vi "34970 Initialize +++.vi"(0 "VISA resource name":refnum<visa-resource-name>, 5 "ID Query (T: Check)":bool=TRUE, 7 "Instr Config":enum16{"no change", "Reset", "Preset"}(ring), 9 "Serial Port Configuration":T1={"Timeout Value (10000)"=10000, "Baud Rate (57600)"=enum."57600", "Flow Control (1:XON / XOFF)"=enum."XON / XOFF"}, 11 "error in (no error)":errorcluster) -> (4 "VISA session":refnum<visa-resource-name>, 15 "error out":errorcluster)   [LabVIEW 2020]
doc: "This VI passes the addressing information for GPIB, or the serial port configuration to the VISA Open VI. You must run this VI before using any of the instrument driver VIs for this instrument.\n\nIt can optionally check the the instrument ID, but error reporting for this still flawed. Modified to allow instrument configuration Reset, Preset(see pp 160, 161 user manual), or No Change.\nW. Gilbert, University of Minnesota Physics, 8/6/2004\nwgilbert@physics.umn.edu"
panel:
  # "See 34970 manual\npp 160,161"
  # "Check\nDon't Check"
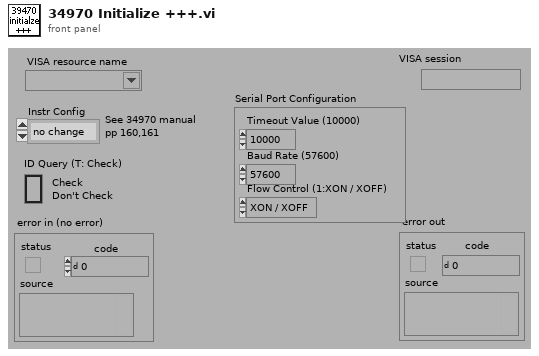
[diagram p1: front panel]
types:
  T1 = cluster{"Timeout Value (10000)":u32, "Baud Rate (57600)":enum16{"1200", "2400", "4800", "9600", "19200", "38400", "57600", "115200"}, "Flow Control (1:XON / XOFF)":enum16{"None", "XON / XOFF", "RTS / CTS", "DTR / DSR"}}
  T2 = enum16{"1200", "2400", "4800", "9600", "19200", "38400", "57600", "115200"}
  T3 = enum16{"None", "XON / XOFF", "RTS / CTS", "DTR / DSR"}
  T4 = cluster{"status":bool, "code":i32, "VI Name":string}
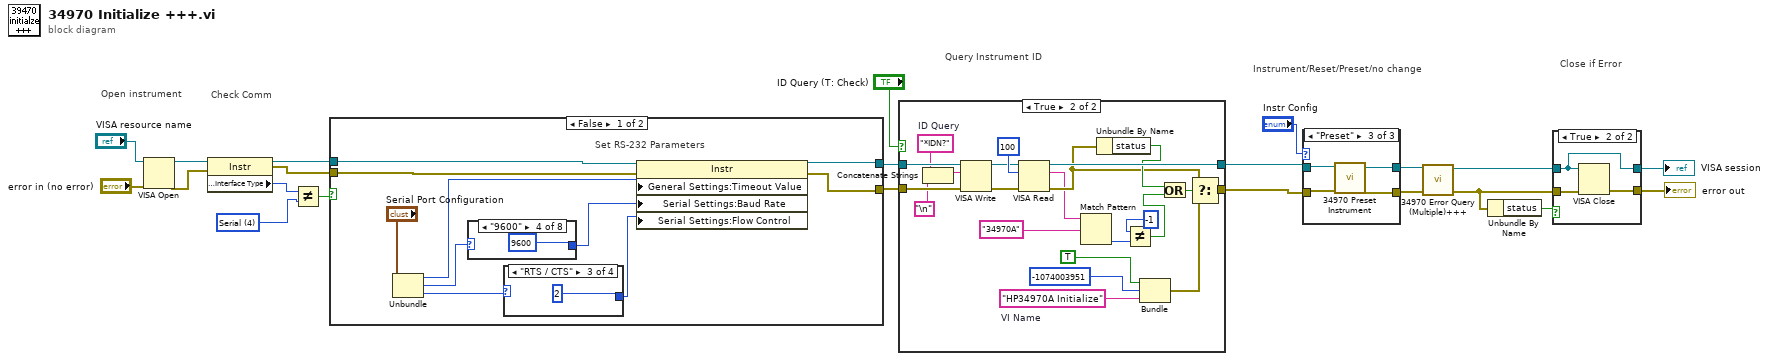
[diagram p0: block diagram]
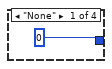
[diagram p2: hidden frame]
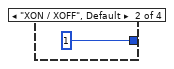
[diagram p3: hidden frame]
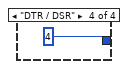
[diagram p4: hidden frame]
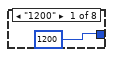
[diagram p5: hidden frame]
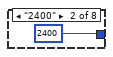
[diagram p6: hidden frame]
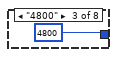
[diagram p7: hidden frame]
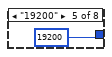
[diagram p8: hidden frame]
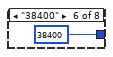
[diagram p9: hidden frame]
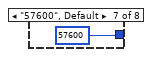
[diagram p10: hidden frame]
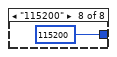
[diagram p11: hidden frame]
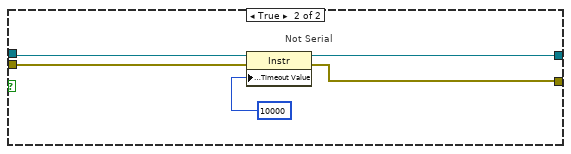
[diagram p12: hidden frame]
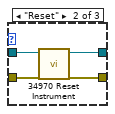
[diagram p15: hidden frame]
diagram:
  w13 = u16 4 items=["GPIB"=1, "VXI"=2, "GPIB-VXI"=3, "Serial"=4, "PXI"=5] ("Interface Information:Interface Type")
  # "Check Comm"
  # "Close if Error"
  # "Query Instrument ID"
  # "Instrument/Reset/Preset/no change"
  # "Open instrument"
  n1 = VISA Open(error in (no error)="error in (no error)", VISA resource name="VISA resource name") -> (VISA resource name=w17:refnum<visa-resource-name>, error out=w14:errorcluster)  [unwired: 1 in, 2 out]
  n2 = property class="Instr"(reference=w17, error in=w14) -> (reference out=w16:refnum<visa-resource-name>, error out=w15:errorcluster, "Interface Information:Interface Type"=w10:u16)
  n3 = Not Equal?(x=w10, y=w13) -> (x != y?=w12:bool)
  n4 = case shown="False" w12 {
    tunnel: [w24 w47] -> w9
    tunnel: w16 -> [w32 w49]
    tunnel: [w23 w45] -> w8
    tunnel: w15 -> [w31 w48]
    frame False {
      # "Set RS-232 Parameters"
      n5 = Unbundle("Serial Port Configuration") -> ("Timeout Value (10000)"=w27:u32, "Baud Rate (57600)"=w29:T2, "Flow Control (1:XON / XOFF)"=w26:T3)
      n6 = case shown="\"9600\"" w29 {
        tunnel: [u32 1200 u32 2400 u32 4800 u32 9600 u32 19200 u32 38400 u32 57600 u32 115200] -> w28
        frame "1200" {
        }
        frame "2400" {
        }
        frame "4800" {
        }
        frame "9600" {
        }
        frame "19200" {
        }
        frame "38400" {
        }
        frame "57600", Default {
        }
        frame "115200" {
        }
      }
      n7 = case shown="\"RTS / CTS\"" w26 {
        tunnel: [0 1 2 4] -> w25
        frame "None" {
        }
        frame "XON / XOFF", Default {
        }
        frame "RTS / CTS" {
        }
        frame "DTR / DSR" {
        }
      }
      n8 = property class="Instr"(reference=w32, error in=w31, "General Settings:Timeout Value"=w27, "Serial Settings:Baud Rate"=w28, "Serial Settings:Flow Control"=w25) -> (reference out=w24:refnum<visa-resource-name>, error out=w23:errorcluster)
    }
    frame True {
      # "Not Serial"
      n9 = property class="Instr"(reference=w49, error in=w48, "General Settings:Timeout Value"=u32 10000 ("Tmo Value")) -> (reference out=w47:refnum<visa-resource-name>, error out=w45:errorcluster)
    }
  }
  n10 = case shown="True" "ID Query (T: Check)" {
    tunnel: [w50 w73] -> w5
    tunnel: [w51 w70] -> w6
    tunnel: w9 -> [w51 w71]
    tunnel: w8 -> [w50 w72]
    frame False {
    }
    frame True {
      w52 = "*IDN?"  # ID Query
      w55 = "HP34970A Initialize"  # VI Name
      n11 = Concatenate Strings(w52, "\n") -> (w53:string)
      n12 = VISA Write(VISA resource name=w71, write buffer=w53, error in (no error)=w72) -> (VISA resource name out=w58:refnum<visa-resource-name>, error out=w60:errorcluster)  [unwired: 1 out]
      n13 = VISA Read(VISA resource name=w58, byte count=u32 100, error in (no error)=w60) -> (VISA resource name out=w70:refnum<visa-resource-name>, read buffer=w57:string, error out=w59:errorcluster)  [unwired: 1 out]
      n14 = Match Pattern(string=w57, regular expression="34970A") -> (offset past match=w65:i32)  [unwired: 4 out]
      n15 = Unbundle By Name(w59) -> ("status"=w62:bool)
      n16 = Not Equal?(x=-1, y=w65) -> (x != y?=w56:bool)
      n17 = Bundle(TRUE, -1074003951, "VI Name"=w55) -> (w67:cluster{bool, i32, "VI Name":string})  [unwired: 1 out]
      n18 = Or(x=w62, y=w56) -> (x .or. y?=w61:bool)
      n19 = Select(t=w59, s=w61, f=w67) -> (s? t:f=w73:T4)
    }
  }
  n20 = case shown="\"Preset\"" "Instr Config" {
    tunnel: w5 -> [w74 w76 w82]
    tunnel: [w74 w79 w80] -> w3
    tunnel: w6 -> [w75 w77 w83]
    tunnel: [w75 w78 w81] -> w4
    frame "no change", Default {
    }
    frame "Reset" {
      n21 = call "34970 Reset Instrument.vi"("VISA resource name"=w77, "error in (no error)"=w76) -> ("VISA resource name out"=w78:refnum<visa-resource-name>, "error out"=w79:errorcluster)  [unwired: 12 in]
    }
    frame "Preset" {
      n22 = call "34970 Preset Instrument.vi"("error in (no error)"=w82, "VISA session"=w83) -> ("error out"=w80:errorcluster, "dup VISA session"=w81:refnum<visa-resource-name>)  [unwired: 8 in]
    }
  }
  n23 = call "34970 Error Query (Multiple)+++.vi"("VISA resource name"=w4, "error in (no error)"=w3) -> ("VISA resource name out"=w2:refnum<visa-resource-name>, "error out"=w1:errorcluster)  [unwired: 10 in, 2 out]
  n24 = Unbundle By Name(w1) -> ("status"=w19:bool)
  n25 = case shown="True" w19 {
    tunnel: w2 -> [w85 w86]
    tunnel: w1 -> [w84 w88]
    tunnel: [w85 w86] -> w18
    tunnel: [w84 w87] -> w11
    frame False {
    }
    frame True {
      n26 = VISA Close(VISA resource name=w86, error in (no error)=w88) -> (error out=w87:errorcluster)
    }
  }
  "VISA session" <- w18
  "error out" <- w11
